vi "Event Create.vi"(8 "error in (no error)":errorcluster, 11 "Event name":string) -> (0 "error out":errorcluster, 3 "Event DVR out":refnum<data-value>)   [LabVIEW 2015, in "MDSplus.lvlib"]
uses:
  MDSplus.lvlib
  Classes/Event_Class/Event.lvclass
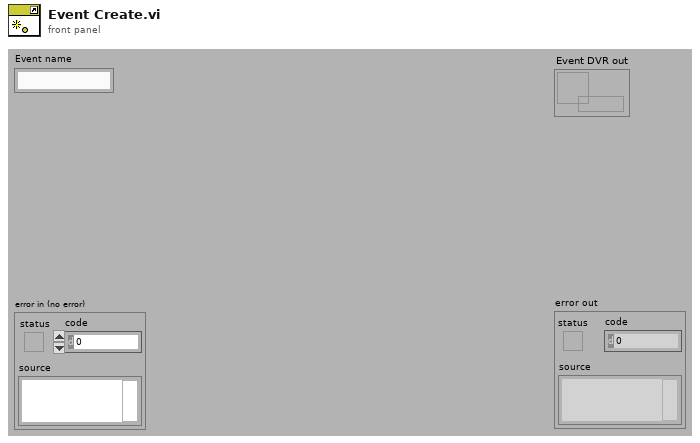
[diagram p1: front panel]
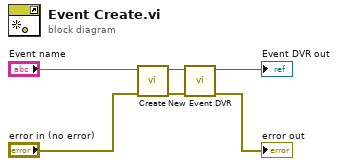
[diagram p0: block diagram]
diagram:
  n1 = call "Create.vi"("error in (no error)"="error in (no error)", "Event name"="Event name") -> ("error out"=w5:errorcluster, "Event out"=w6:refnum<class "Event.lvclass">)  [unwired: 8 in]
  n2 = call "New Event DVR.vi"("error in (no error)"=w5, "Event in"=w6) -> ("error out"=→"error out":errorcluster, "Event DVR out"=→"Event DVR out":refnum<data-value>)  [unwired: 8 in]
